vi "Color Table Generator.vi"() -> (0 "?":u32[](array[colorbox]))   [LabVIEW 2012]
doc: "Color Table Generator.vi是Color Table Example.vi的子VI。\n\n依据用户指定的初始、中间和最终RGB颜色生成色码表。通过波形图和游标，用户可通过红色、绿色和蓝色创建色码表的开始、中间、结束颜色。\n\n通过Component Generator.vi计算标尺。更多信息见子VI的说明信息。"
panel:
  in  "Less Than 0":u32(colorbox) caption="小于0？"
  in  "MoreThan 255":u32(colorbox)=16711680 caption="大于255"
  in  "Cancel":bool caption="取消"
  in  "Accept":bool caption="接受"
  in  "final color":cluster{u8, u8, u8}(slide)={255, 234, 0} caption="最终颜色" scale=0.0..255.0
  in  "beginning color":cluster{u8, u8, u8}(slide)={0, 21, 255} caption="开始颜色" scale=0.0..255.0
  out "?":cluster{"Component Array":u32[]}[](graph)
  # "依据用户指定的初始、中间和最终RGB颜色生成色码表。通过滑块指定RGB标尺的初始颜色和最终颜色。通过游标定义中间颜色。"
  # "更多信息，见“文件>>VI属性>>说明信息”。"
  # "值大于255时，超出颜色范围。"
  # "值小于0时，超出颜色范围。"
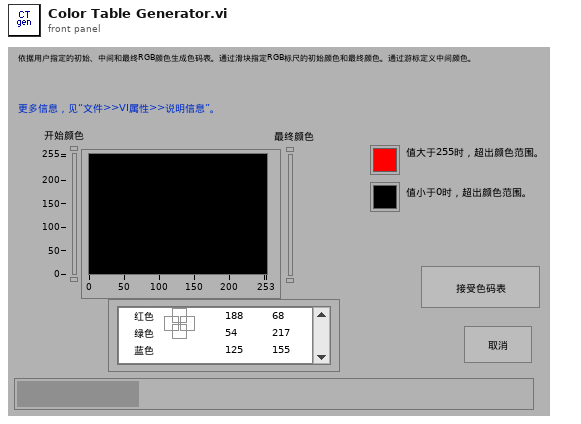
[diagram p1: front panel]
types:
  T1 = cluster{u8, u8, "Cursor.Cursor Y":dbl, "Cursor.Cursor X":dbl}
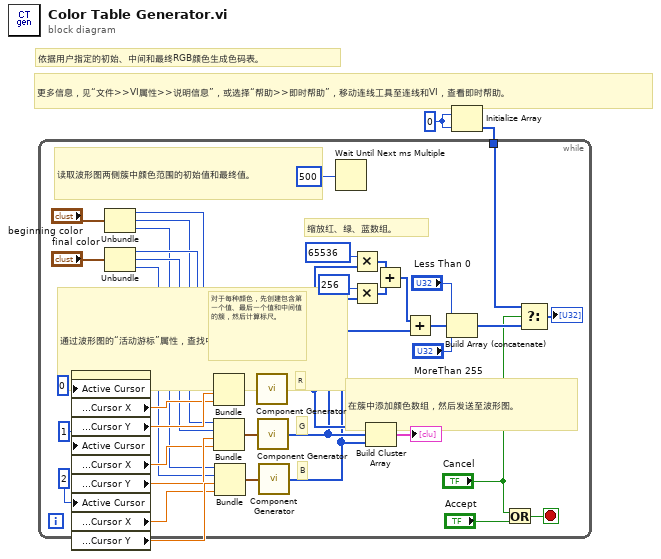
[diagram p0: block diagram]
diagram:
  w2 = u32 0
  # "依据用户指定的初始、中间和最终RGB颜色生成色码表。"
  # "更多信息，见“文件>>VI属性>>说明信息”，或选择“帮助>>即时帮助”，移动连线工具至连线和VI，查看即时帮助。"
  n1 = Initialize Array(w2, w2) -> (w1:u32[])
  n2 = while {
    tunnel: w1 -> [w17]
    stop <- w18 stop-if-true
    # "对于每种颜色，先创建包含第一个值、最后一个值和中间值的簇，然后计算标尺。"
    # "缩放红、绿、蓝数组。"
    # "在簇中添加颜色数组，然后发送至波形图。"
    # "通过波形图的“活动游标”属性，查找中点的位置和值。"
    # "读取波形图两侧簇中颜色范围的初始值和最终值。"
    # "B"
    # "G"
    # "R"
    n3 = property class="WFGraph (严格)"("Active Cursor"=0, "Active Cursor"=1, "Active Cursor"=2) -> ("Cursor.Cursor Position:Cursor X"=w36:dbl, "Cursor.Cursor Position:Cursor Y"=w37:dbl, "Cursor.Cursor Position:Cursor X"=w38:dbl, "Cursor.Cursor Position:Cursor Y"=w39:dbl, "Cursor.Cursor Position:Cursor X"=w40:dbl, "Cursor.Cursor Position:Cursor Y"=w41:dbl)  [unwired: 2 in, 2 out]
    n4 = Unbundle("beginning color") -> (w30:u8, w31:u8, w32:u8)
    n5 = Unbundle("final color") -> (w33:u8, w34:u8, w35:u8)
    n6 = Bundle(w30, w33, "Cursor.Cursor Y"=w37, "Cursor.Cursor X"=w36) -> (w27:T1)  [unwired: 1 in]
    n7 = Bundle(w31, w34, "Cursor.Cursor Y"=w39, "Cursor.Cursor X"=w38) -> (w14:T1)  [unwired: 1 in]
    n8 = Bundle(w32, w35, "Cursor.Cursor Y"=w41, "Cursor.Cursor X"=w40) -> (w13:T1)  [unwired: 1 in]
    n9 = call "Component Generator.vi"("Component definition"=w27) -> ("Component Array"=w5:u32[])
    n10 = call "Component Generator.vi"("Component definition"=w14) -> ("Component Array"=w4:u32[])
    n11 = call "Component Generator.vi"("Component definition"=w13) -> ("Component Array"=w3:u32[])
    n12 = Wait Until Next ms Multiple(millisecond multiple=500) -> ()  [unwired: 1 out]
    n13 = Multiply(x=u32 65536, y=w5) -> (x*y=w22:u32[])
    n14 = Multiply(x=u32 256, y=w4) -> (x*y=w21:u32[])
    n15 = Build Cluster Array(w5, w4, w3) -> (→"?":cluster{"Component Array":u32[]}[])
    n16 = Add(x=w22, y=w21) -> (x+y=w23:u32[])
    n17 = Add(x=w23, y=w3) -> (x+y=w9:u32[])
    n18 = Build Array (concatenate)("Less Than 0", w9, "MoreThan 255") -> (w12:u32[])
    n19 = Or(x="Cancel", y="Accept") -> (x .or. y?=w18:bool)
    n20 = Select(t=w17, s="Cancel", f=w12) -> (s? t:f=→"?":u32[])
  }
